vi "offset.set.vi"(8 "error in (no error)":errorcluster, 10 "offset":timestamp format="%<%x %.3X>T", 11 "ts.relative in":refnum<class "ts.relative.lvclass">) -> (0 "error out":errorcluster, 3 "ts.relative out":refnum<class "ts.relative.lvclass">)   [LabVIEW 2020, in "ts.relative.lvclass"]
uses:
  ts.relative.lvclass
  ts.relative.lvclass/ts.relative.ctl
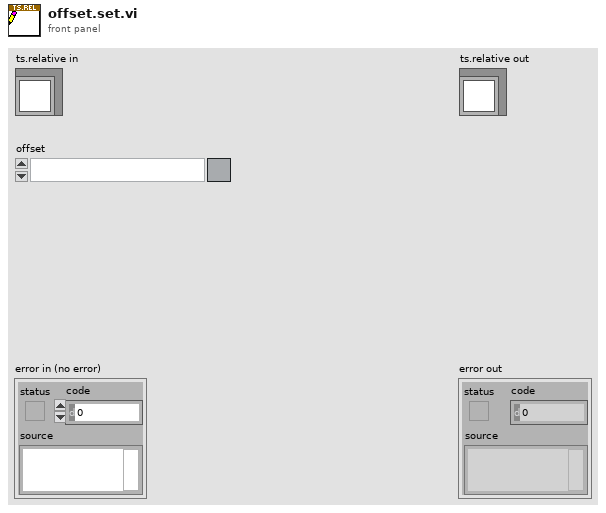
[diagram p1: front panel]
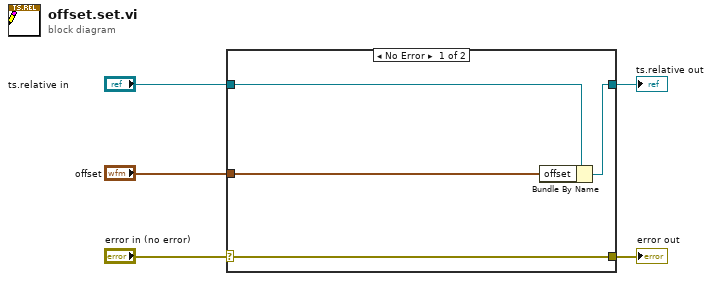
[diagram p0: block diagram]
diagram:
  n1 = case shown="No Error" "error in (no error)" {
    selector: "error in (no error)" -> [w9 w10]
    tunnel: [w9 w10] -> w4
    tunnel: [w7 w11] -> w2
    tunnel: "ts.relative in" -> [w8 w11]
    tunnel: "offset" -> [w6 _]
    frame No Error {
      n2 = Bundle By Name(cluster=w8, "offset"=w6) -> (w7:refnum<class "ts.relative.lvclass">)
    }
    frame Error {
    }
  }
  "error out" <- w4
  "ts.relative out" <- w2
